vi "init.vi"(8 "error in (no error)":errorcluster, 9 "Port":u16, 10 "IP":string="140.252.32.237", 11 "Mockbus in":refnum<class "Mockbus.lvclass">) -> (0 "error out":errorcluster, 3 "Mockbus out":refnum<class "Mockbus.lvclass">)   [LabVIEW 2015, in "Mockbus.lvclass"]
uses:
  Mockbus.lvclass
  Mockbus.lvclass/Mockbus.ctl
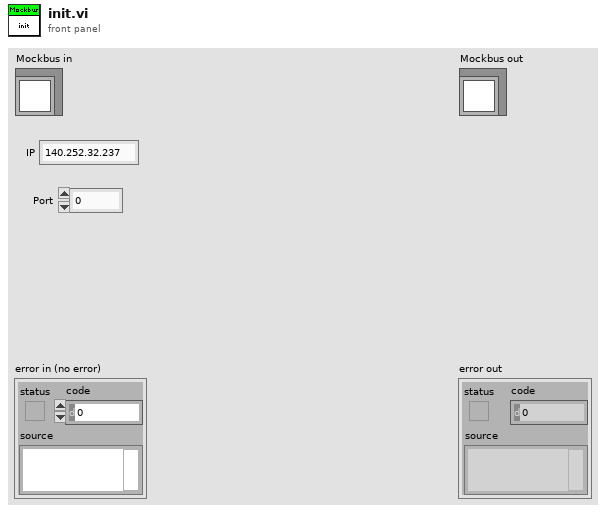
[diagram p1: front panel]
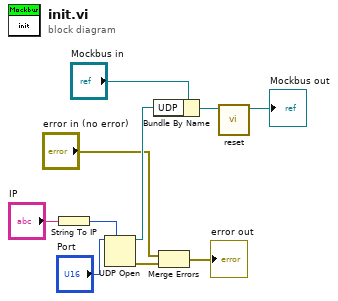
[diagram p0: block diagram]
diagram:
  n1 = String To IP(1:"IP") -> (0:w9:u32)
  n2 = UDP Open(7:w9, 11:"Port") -> (port=w6:refnum<k16>, 0:w4:errorcluster)  [unwired: 3 in, 1 out]
  n3 = Bundle By Name(cluster="Mockbus in", "UDP"=w6) -> (w2:refnum<class "Mockbus.lvclass">)
  n4 = Merge Errors("error in (no error)", w4) -> (→"error out":errorcluster)
  n5 = call "reset.vi"("Mockbus in"=w2) -> ("Mockbus out"=→"Mockbus out":refnum<class "Mockbus.lvclass">)  [unwired: 9 in, 1 out]
